vi "Detect Intake Object.vi"(11 "Refnum in":T2(plugin-control)) -> (0 "Object Found?":bool, 1 "Object Type":T1, 3 "Refnum out":T2(plugin-control))   [LabVIEW 2014]
uses:
  2015 Crabby Code/Common Code/Elevator Object Type.ctl
  <vilib>/vision/NI_Vision_Development_Module.lvlib
panel:
  in  "Zone Size":dbl=7.0 format="%#_13g"
  in  "Sat Thresh":dbl
  in  "Luma Thresh":dbl
  out "Sat":dbl format="%.6f"
  out "Luma":dbl format="%.6f"
  out "Avg Hue":bool
  out "B":dbl
  out "G":dbl
  out "Avg Color":bool
  out "R":dbl
  out "Red or Hue Plane out":T2(plugin-control)
  in  "Exam Zone Offset Y":dbl
  in  "Exam Zone Offset X":dbl
  out "Image Dst Out":T2(plugin-control)
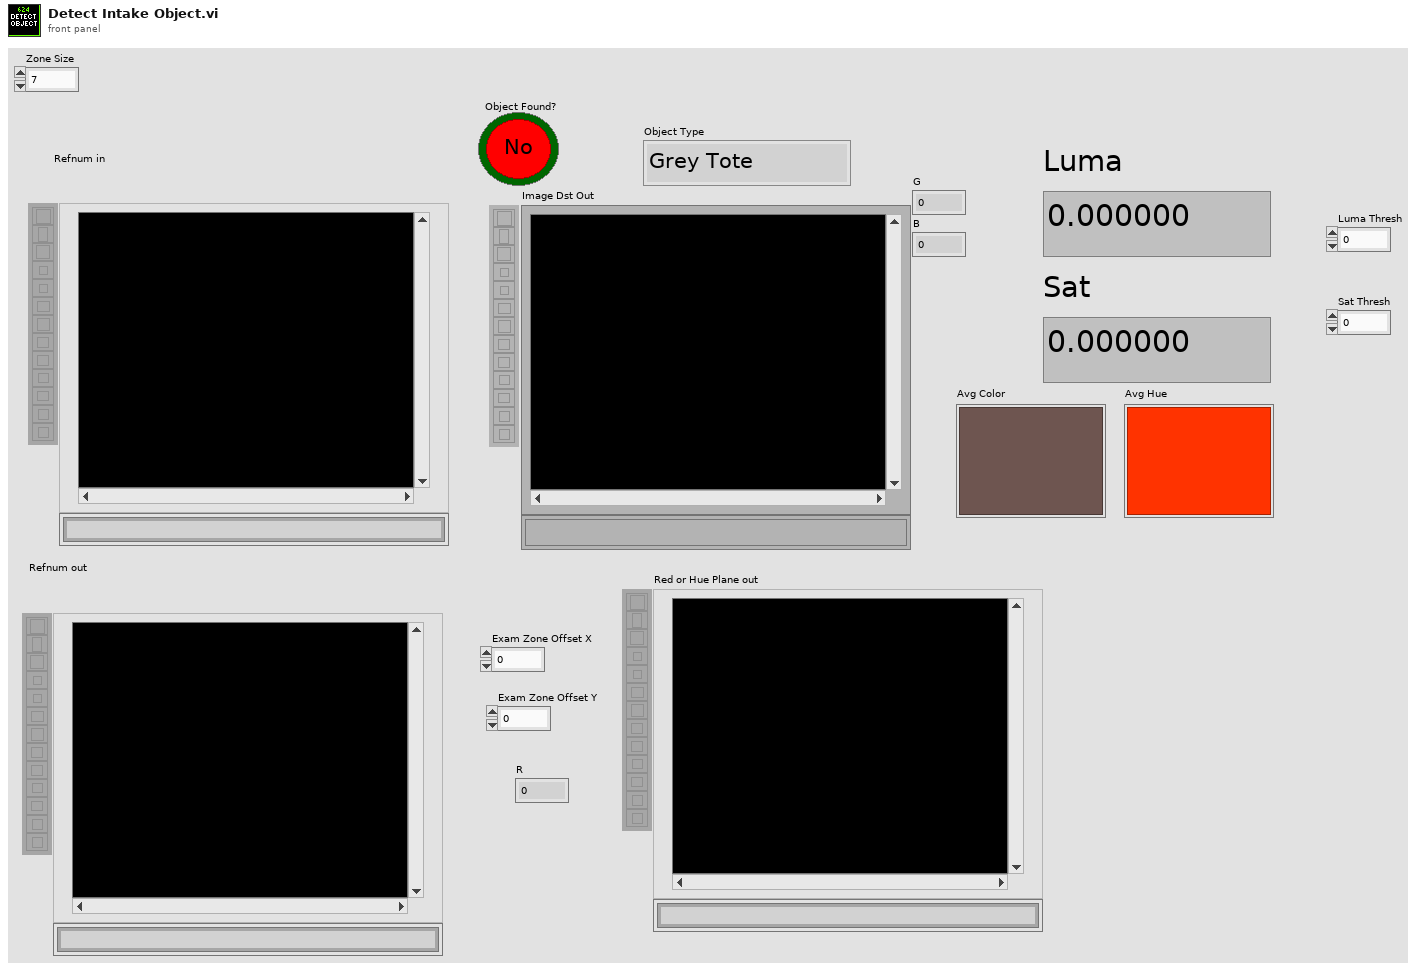
[diagram p1: front panel]
types:
  T1 = typedef "Elevator Object Type.ctl" = enum16{"Grey Tote", "Yellow Tote", "Trash Can"}
  T2 = typedef "IMAQ Image.ctl" = refnum<image>
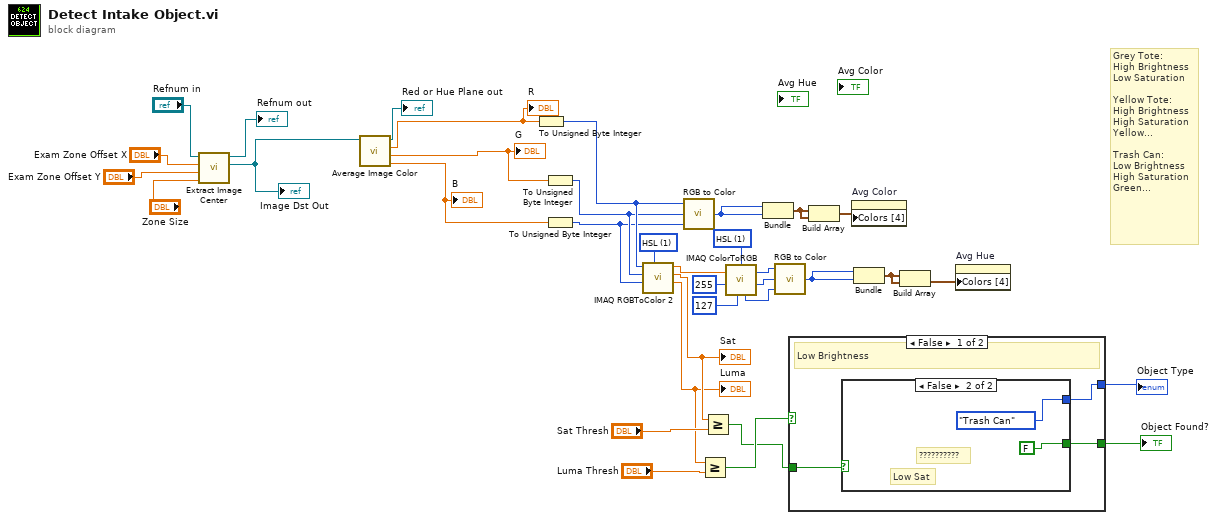
[diagram p0: block diagram]
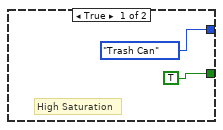
[diagram p2: hidden frame]
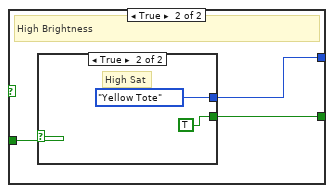
[diagram p3: hidden frame]
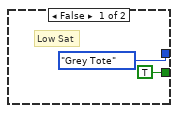
[diagram p4: hidden frame]
diagram:
  w19 = u16 1 items=["RGB", "HSL", "HSV", "HSI"] ("Color Mode")
  w20 = u16 1 items=["RGB", "HSL", "HSV", "HSI", "CIE L*a*b*", "CIE XYZ"] ("Color Mode")
  # "Grey Tote:\nHigh Brightness\nLow Saturation\n\nYellow Tote:\nHigh Brightness\nHigh Saturation\nYellow...\n\nTrash Can:\nLow Brightness\nHigh Saturation\nGreen..."
  n1 = call "Extract Image Center.vi"("Zone Size"="Zone Size", "Exam Zone Offset Y"="Exam Zone Offset Y", "Exam Zone Offset X"="Exam Zone Offset X", "Source In"="Refnum in") -> ("Extracted Out"=w31:T2, "Annotated Source Out"=→"Refnum out":T2)  [unwired: 6 in]
  "Image Dst Out" <- w31
  n2 = call "Average Image Color.vi"("Refnum in"=w31) -> ("B"=w9:dbl, "G"=w26:dbl, "R"=w29:dbl, "Refnum out"=→"Red or Hue Plane out":T2)  [unwired: 7 in]
  "R" <- w29
  "G" <- w26
  "B" <- w9
  n3 = To Unsigned Byte Integer(number=w29) -> (unsigned 8bit integer=w24:u8)
  n4 = To Unsigned Byte Integer(number=w26) -> (unsigned 8bit integer=w23:u8)
  n5 = To Unsigned Byte Integer(number=w9) -> (unsigned 8bit integer=w22:u8)
  n6 = call "IMAQ RGBToColor 2"("Color Mode"=w20, "Blue value"=w22, "Green value"=w23, "Red value"=w24) -> ("Blue or Luma or Val or Inten or Z or b*value"=w6:dbl, "Green or Sat or Y or a* value"=w8:dbl, "Red or Hue or X or L* value"=w21:dbl)  [unwired: 4 in, 1 out]
  "Luma" <- w6
  "Sat" <- w8
  n7 = call <vilib>:"RGB to Color.vi"("B"=w22, "G"=w23, "R"=w24) -> ("Color"=w25:u32)
  n8 = Greater Or Equal?(x=w6, y="Luma Thresh") -> (x >= y?=w2:bool)
  n9 = Greater Or Equal?(x=w8, y="Sat Thresh") -> (x >= y?=w1:bool)
  n10 = call "IMAQ ColorToRGB"("Green or Sat value"=u8 255, "Blue or Luma or Val or Inten value"=u8 127, "Red or Hue value"=w21, "Color Mode"=w19) -> ("Blue value"=w12:u8, "Green value"=w13:u8, "Red value"=w14:u8)  [unwired: 1 in, 1 out]
  n11 = Bundle("Color"=w25, "Color"=w25) -> (w28:cluster{"Color":u32, "Color":u32})  [unwired: 1 in]
  n12 = call <vilib>:"RGB to Color.vi"("B"=w12, "G"=w13, "R"=w14) -> ("Color"=w16:u32)
  n13 = case shown="False" w2 {
    tunnel: [w37 w43] -> w4
    tunnel: w1 -> [w38 w45]
    tunnel: [w36 w44] -> w3
    frame False {
      # "Low Brightness"
      n14 = case shown="False" w38 {
        tunnel: [Elevator_Object_Type."Trash Can" Elevator_Object_Type."Trash Can"] -> w37
        tunnel: [TRUE FALSE] -> w36
        frame True {
          # "High Saturation"
        }
        frame False {
          # "??????????"
          # "Low Sat"
        }
      }
    }
    frame True {
      # "High Brightness"
      n15 = case shown="True" w45 {
        tunnel: [TRUE TRUE] -> w44
        tunnel: [Elevator_Object_Type."Grey Tote" Elevator_Object_Type."Yellow Tote"] -> w43
        frame False {
          # "Low Sat"
        }
        frame True {
          # "High Sat"
        }
      }
    }
  }
  "Object Type" <- w4
  "Object Found?" <- w3
  n16 = Build Array(w28, w28) -> (w27:cluster{"Color":u32, "Color":u32}[])
  n17 = property on="Avg Color" class="Bool (strict)"("Colors [4]"=w27) -> ()  [unwired: 2 in, 2 out]
  n18 = Bundle("Color"=w16, "Color"=w16) -> (w15:cluster{"Color":u32, "Color":u32})  [unwired: 1 in]
  n19 = Build Array(w15, w15) -> (w11:cluster{"Color":u32, "Color":u32}[])
  n20 = property on="Avg Hue" class="Bool (strict)"("Colors [4]"=w11) -> ()  [unwired: 2 in, 2 out]
